vi "GUNSC_Str2EXtensions.v.vi"(8 "error in":errorcluster, 10 "command":string, 11 "max amps":u16=128) -> (0 "error IO":errorcluster, 2 "Extensions":u16[](array[numeric]))   [LabVIEW 2016]
panel:
  out "output array":i32[](array[numeric])
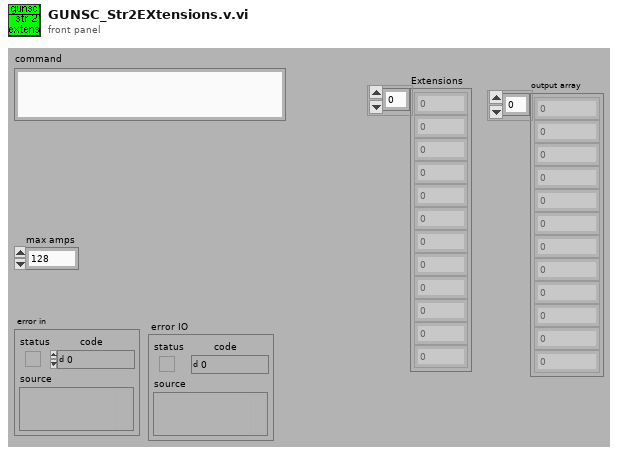
[diagram p1: front panel]
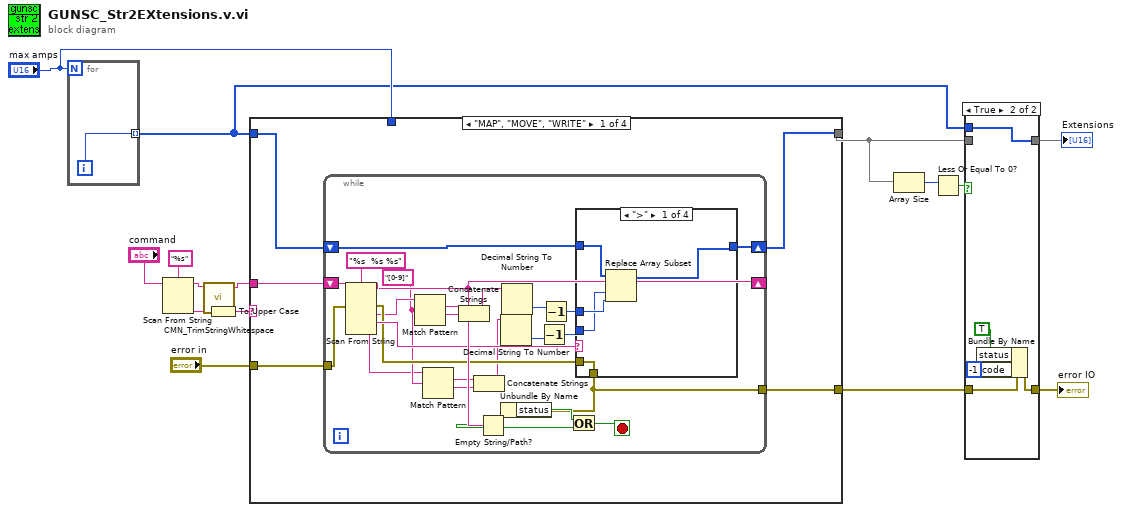
[diagram p0: block diagram]
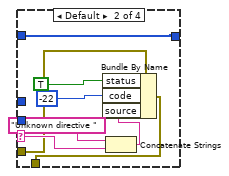
[diagram p3: hidden frame]
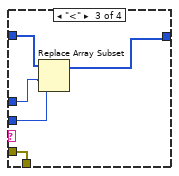
[diagram p4: hidden frame]
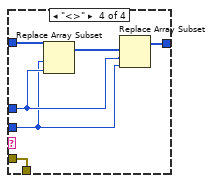
[diagram p5: hidden frame]
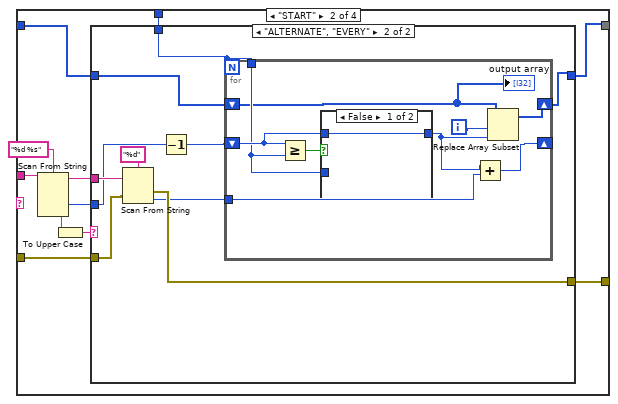
[diagram p6: hidden frame]
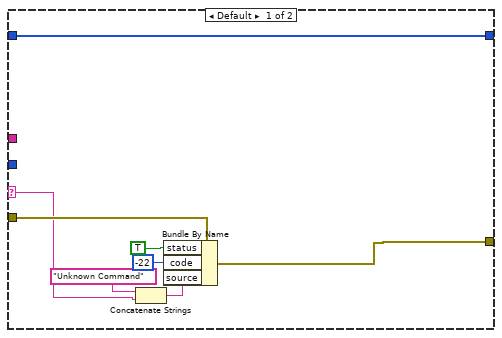
[diagram p7: hidden frame]
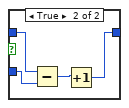
[diagram p8: hidden frame]
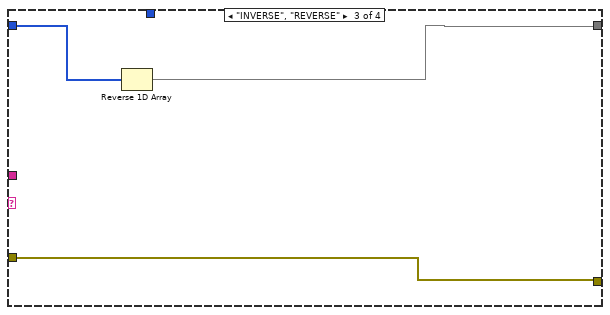
[diagram p9: hidden frame]
diagram:
  n1 = for {
    N: "max amps" -> [_]
    tunnel: [w16] -> w1 mode=indexing
    i -> [w16]
  }
  n2 = Scan From String(format string="%s", input string="command") -> (remaining string=w10:string, output 1=w13:string)  [unwired: 2 in, 3 out]
  n3 = call "CMN_TrimStringWhitespace.vi"("string"=w10) -> ("trimmed string"=w9:string)  [unwired: 1 in, 8 out]
  n4 = To Upper Case(1:w13) -> (0:w12:string)
  n5 = case shown="\"MAP\", \"MOVE\", \"WRITE\"" w12 {
    tunnel: w9 -> [w17 w81 _ _]
    tunnel: w1 -> [w21 w73 w116 w118]
    tunnel: [w20 w72 w115 w118] -> w3
    tunnel: "error in" -> [w19 w75 w114 w117]
    tunnel: [w18 w74 w114 w117] -> w5
    tunnel: "max amps" -> [_ w71 _ _]
    frame "MAP", "MOVE", "WRITE" {
      n6 = while {
        shift-right: [w44] -> _
        shift-left: w17 -> [w46]
        shift-right: [w43] -> w20
        shift-left: w21 -> [w39]
        tunnel: w19 -> [w35]
        tunnel: [w33] -> w18
        stop <- w36 stop-if-true
        w27 = "[0-9]" ("regular expression")
        n7 = Scan From String(format string="%s  %s %s", input string=w46, error in=w35) -> (remaining string=w44:string, error out=w34:errorcluster, output 1=w32:string, output 2=w40:string, output 3=w26:string)  [unwired: 1 in, 4 out]
        n8 = Match Pattern(string=w32, regular expression=w27) -> (match substring=w31:string, after substring=w30:string)  [unwired: 3 out]
        n9 = Match Pattern(string=w26, regular expression=w27) -> (match substring=w25:string, after substring=w24:string)  [unwired: 3 out]
        n10 = Concatenate Strings(w31, w30) -> (w29:string)
        n11 = Concatenate Strings(w25, w24) -> (w23:string)
        n12 = Empty String/Path?(string/path=w44) -> (empty?=w38:bool)
        n13 = Decimal String To Number(string=w23) -> (number=w22:i32)  [unwired: 3 out]
        n14 = Decimal String To Number(string=w29) -> (number=w28:i32)  [unwired: 3 out]
        n15 = Decrement(x=w22) -> (x-1=w42:i32)
        n16 = Decrement(x=w28) -> (x-1=w41:i32)
        n17 = case shown="\">\"" w40 {
          selector: w40 -> [_ w55 _ _]
          tunnel: [w50 w59 w63 w70] -> w43
          tunnel: w42 -> [w48 _ w61 w66]
          tunnel: w41 -> [w49 _ w62 w67]
          tunnel: w39 -> [w51 w59 w64 w69]
          tunnel: w34 -> [w47 w53 w60 w65]
          tunnel: [w47 w52 w60 w65] -> w33
          frame ">" {
            n18 = Replace Array Subset(array=w51, new element=w49, index=w48) -> (w50:i32[])
          }
          frame Default {
            n19 = Concatenate Strings("Unknown directive " ("source"), w55) -> (w54:string)
            n20 = Bundle By Name(cluster=w53, "status"=TRUE, "code"=-22, "source"=w54) -> (w52:errorcluster)
          }
          frame "<" {
            n21 = Replace Array Subset(array=w64, new element=w61, index=w62) -> (w63:i32[])
          }
          frame "<>" {
            n22 = Replace Array Subset(array=w69, new element=w67, index=w66) -> (w68:i32[])
            n23 = Replace Array Subset(array=w68, new element=w66, index=w67) -> (w70:i32[])
          }
        }
        n24 = Unbundle By Name(w33) -> ("status"=w37:bool)
        n25 = Or(x=w37, y=w38) -> (x .or. y?=w36:bool)
      }
    }
    frame "START" {
      n26 = Scan From String(format string="%d %s", input string=w81) -> (remaining string=w76:string, output 1=w77:i32, output 2=w79:string)  [unwired: 2 in, 4 out]
      n27 = To Upper Case(1:w79) -> (0:w78:string)
      n28 = case shown="\"ALTERNATE\", \"EVERY\"" w78 {
        selector: w78 -> [w85 _]
        tunnel: w77 -> [_ w92]
        tunnel: w76 -> [_ w99]
        tunnel: w75 -> [w89 w97]
        tunnel: [w83 w96] -> w74
        tunnel: w73 -> [w82 w90]
        tunnel: [w82 w94] -> w72
        tunnel: w71 -> [_ w93]
        frame Default {
          n29 = Concatenate Strings("Unknown Command" ("source"), w85) -> (w84:string)
          n30 = Bundle By Name(cluster=w89, "status"=TRUE, "code"=-22, "source"=w84) -> (w83:errorcluster)
        }
        frame "ALTERNATE", "EVERY" {
          n31 = Scan From String(format string="%d", input string=w99, error in=w97) -> (error out=w96:errorcluster, output 1=w95:i32)  [unwired: 1 in, 3 out]
          n32 = Decrement(x=w92) -> (x-1=w91:i32)
          n33 = for {
            N: w93 -> [_]
            shift-right: [w103] -> w94
            shift-left: w90 -> [w102]
            tunnel: w95 -> [w108]
            tunnel: w93 -> [w104]
            shift-right: [w107] -> _
            shift-left: w91 -> [w106]
            i -> [w101]
            n34 = Greater Or Equal?(x=w106, y=w104) -> (x >= y?=w105:bool)
            n35 = case shown="False" w105 {
              tunnel: w106 -> [w109 w111]
              tunnel: [w109 w112] -> w100
              tunnel: w104 -> [_ w110]
              frame False {
              }
              frame True {
                n36 = Subtract(x=w111, y=w110) -> (x-y=w113:i32)
                n37 = Increment(x=w113) -> (x+1=w112:i32)
              }
            }
            n38 = Add(x=w100, y=w108) -> (x+y=w107:i32)
            n39 = Replace Array Subset(array=w102, new element=w100, index=w101) -> (w103:i32[])
            "output array" <- w102
          }
        }
      }
    }
    frame "INVERSE", "REVERSE" {
      n40 = Reverse 1D Array(array=w116) -> (reversed array=w115:i32[])
    }
    frame "ORDERED", Default {
    }
  }
  n41 = Array Size(array=w3) -> (size(s)=w7:i32)
  n42 = Less Or Equal To 0?(x=w7) -> (x <= 0?=w6:bool)
  n43 = case shown="True" w6 {
    tunnel: w5 -> [w120 w123]
    tunnel: [w120 w122] -> w4
    tunnel: w3 -> [w119 _]
    tunnel: [w119 w121] -> w2
    tunnel: w1 -> [_ w121]
    frame False {
    }
    frame True {
      n44 = Bundle By Name(cluster=w123, "status"=TRUE, "code"=-1) -> (w122:errorcluster)
    }
  }
  "Extensions" <- w2
  "error IO" <- w4
